vi "Oven Average of all temp.vi"() -> ()   [LabVIEW 2013, in "Generic Data Logger.lvlib" / "Fluke 2625A (Hydra II).lvlib" / "Fluke 2625A (Hydra II).lvclass"]
uses:
  Fluke 2625A (Hydra II).lvclass
  <vilib>/express/express shared/transition.llb/Dynamic To Waveform Array.vi
  <vilib>/express/express signal manip/GetorSetDDTAttributes/Set DDT Attributes/SetT0.vi
  <vilib>/express/express shared/transition.llb/Waveform Array To Dynamic.vi
  <vilib>/express/express signal manip/GetorSetDDTAttributes/Set DDT Attributes/Set DDT Properties.xnode
  <instrlib>/Fluke 2625A/Fluke 2625A.lvlib
  Data Logger/Data Logger.lvclass
panel:
  out "time delay":dbl
  out "min length":i32
  out "size(s) 2":i32
  out "before write":errorcluster
  out "error out":errorcluster
  out "Path":string
  out "selected path":path
  out "Current Average":dbl
  out "addign all values":dbl
  out "size(s)":i32
  out "length of stuff":i32
  out "String Array":string[](array[string])
  out "i":i32
  out "Numeric Array":dbl[](array[numeric])
  out "Raw String":string
  in  "Stop Button":bool
  in  "VISA resource name":refnum<visa-resource-name>
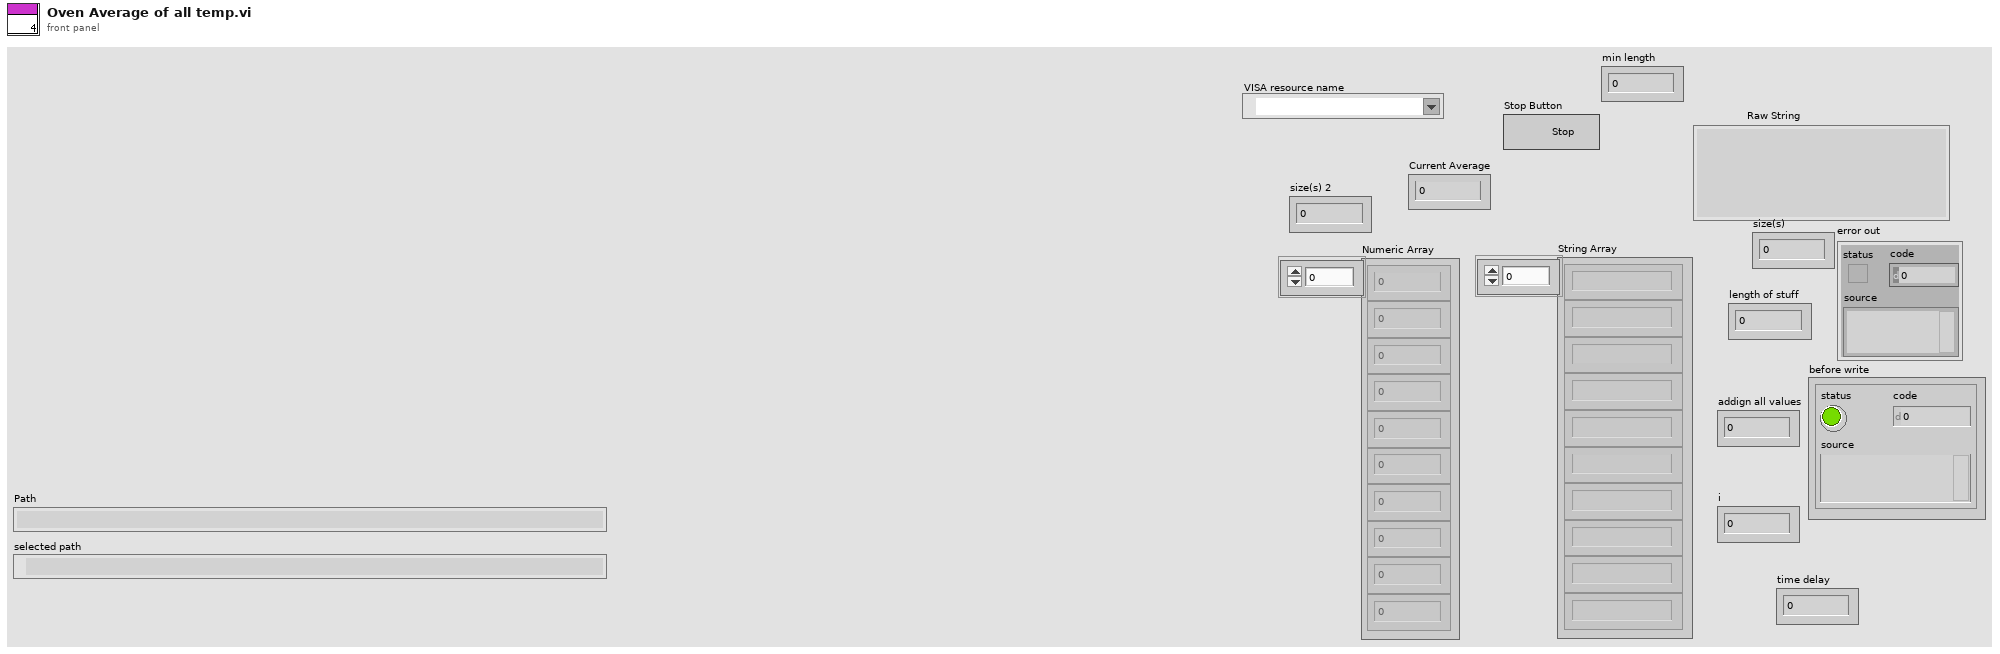
[diagram p1: front panel]
types:
  T1 = cluster{"Project Number":string, "Manufacturer":string, "Model":string, "Serial":string, "Comment":string}
  T2 = typedef "Generic Data Logger.lvlib/Fluke 2625A (Hydra II).lvlib/Fluke 2625A (Hydra II).lvclass/Unit Measurement.ctl" = cluster{"Function (5: Temp)":u16, "Channel":i8, "Thermocouple Type (0: J) 2":u16, "Name":string}
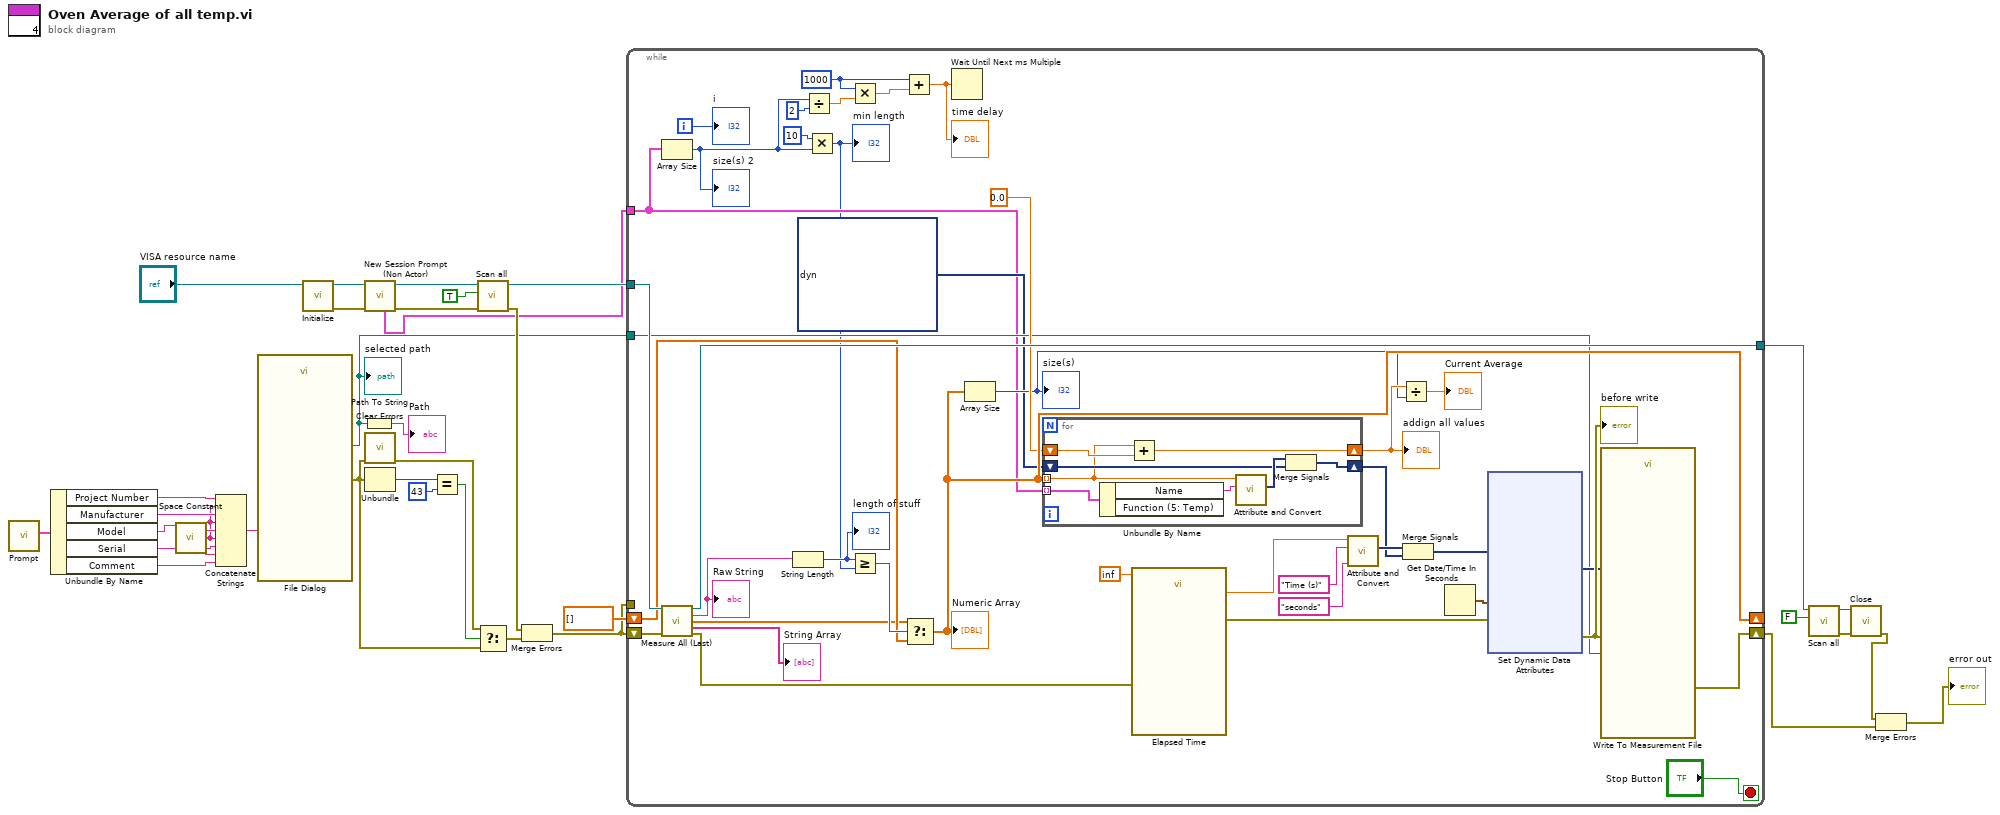
[diagram p0: block diagram]
diagram:
  n1 = call "Prompt.vi"() -> ("Cluster"=w26:T1)  [unwired: 11 in]
  n2 = Unbundle By Name(w26) -> ("Project Number"=w25:string, "Manufacturer"=w24:string, "Model"=w23:string, "Serial"=w22:string, "Comment"=w21:string)
  n3 = call <vilib>:"Space Constant.vi"() -> ("String"=w20:string)
  n4 = Concatenate Strings(w25, w20, w24, w20, w23, w20, w22, w20, w21) -> (w19:string)
  n5 = call "File Dialog"("default name"=w19) -> ("selected path"=w10:path, "error out"=w13:errorcluster)  [unwired: 11 in, 2 out]
  "selected path" <- w10
  n6 = call <instrlib>:"Initialize.vi"("VISA resource name"="VISA resource name") -> ("error out"=w33:errorcluster, "VISA resource name out"=w34:refnum<visa-resource-name>)  [unwired: 8 in, 1 out]
  n7 = Path To String(path=w10) -> (string=→"Path":string)
  n8 = call "New Session Prompt (Non Actor).vi"("error in (no error)"=w33, "VISA resource name"=w34) -> ("error out"=w29:errorcluster, "VISA resource name out"=w30:refnum<visa-resource-name>, "Array 2"=w9:T2[])  [unwired: 5 in, 2 out]
  n9 = call <vilib>:"Clear Errors.vi"("error in (no error)"=w13) -> ("error out"=w14:errorcluster)  [unwired: 6 in]
  n10 = Unbundle(w13) -> ("code"=w17:i32)  [unwired: 2 out]
  n11 = Equal?(x=w17, y=43) -> (x = y?=w15:bool)
  n12 = call <instrlib>:"Scan all.vi"("error in (no error)"=w29, "Start/Stop"=TRUE, "VISA resource name"=w30) -> ("error out"=w12:errorcluster, "VISA resource name out"=w28:refnum<visa-resource-name>)  [unwired: 7 in]
  n13 = Select(t=w14, s=w15, f=w13) -> (s? t:f=w11:errorcluster)
  n14 = Merge Errors(w12, w11) -> (w4:errorcluster)
  n15 = while {
    tunnel: w28 -> [w74]
    tunnel: w4 -> [_]
    tunnel: [w73] -> w6
    shift-right: [w65] -> _
    shift-left: dbl[] [] ("Numeric Array") -> [w66]
    tunnel: w10 -> [w54]
    tunnel: w9 -> [w43]
    shift-right: [w55] -> w2
    shift-left: w4 -> [w45]
    i -> [w71]
    stop <- "Stop Button" stop-if-true
    w37 = u32 1000 ("millisecond multiple")
    n16 = Array Size(array=w43) -> (size(s)=w40:i32)
    "size(s) 2" <- w40
    n17 = call <instrlib>:"Measure All (Last).vi"("VISA resource name out"=w74, "error in (no error)"=w45) -> ("VISA resource name out 2"=w73:refnum<visa-resource-name>, "Raw String"=w69:string, "Numeric Array"=w44:dbl[], "String Array"=→"String Array":string[], "error out 2"=w51:errorcluster)  [unwired: 9 in]
    "Raw String" <- w69
    n18 = String Length(string=w69) -> (length=w68:i32)
    "length of stuff" <- w68
    n19 = Divide(x=w40, y=2) -> (x/y=w36:dbl)
    n20 = Multiply(x=10 ("y"), y=w40) -> (x*y=w41:i32)
    "min length" <- w41
    n21 = Multiply(x=w37, y=w36) -> (x*y=w35:dbl)
    n22 = Greater Or Equal?(x=w68, y=w41) -> (x >= y?=w67:bool)
    n23 = Add(x=w37, y=w35) -> (x+y=w38:dbl)
    "time delay" <- w38
    n24 = Select(t=w44, s=w67, f=w66) -> (s? t:f=w65:dbl[])
    "Numeric Array" <- w65
    n25 = Wait Until Next ms Multiple(millisecond multiple=w38) -> ()  [unwired: 1 out]
    n26 = Array Size(array=w65) -> (size(s)=w62:i32)
    "size(s)" <- w62
    n27 = for {
      tunnel: w65 -> [w89] mode=indexing
      shift-right: [w90] -> w63
      shift-left: 0.0 ("read buffer") -> [w91]
      tunnel: w43 -> [w96] mode=indexing
      shift-right: [w92] -> w47
      shift-left: dynamicdata [] ("Waveform Graph") -> [w93]
      n28 = Unbundle By Name(w96) -> ("Name"=w95:string)  [unwired: 1 out]
      n29 = Add(x=w89, y=w91) -> (x+y=w90:dbl)
      n30 = call "Attribute and Convert.vi"("Signal Name"=w95, "Number in"=w89) -> ("Dynamic Signal Out"=w94:dynamicdata)  [unwired: 9 in]
      n31 = Merge Signals(w94, w93) -> (w92:dynamicdata)
    }
    "addign all values" <- w63
    n32 = call "Elapsed Time"("Time Target (s)"=inf, "error in (no error)"=w51) -> ("Elapsed Time (s)"=w52:dbl, "error out"=w50:errorcluster)  [unwired: 10 in, 6 out]
    n33 = call "Attribute and Convert.vi"("Unit"="seconds", "Signal Name"="Time (s)", "Number in"=w52) -> ("Dynamic Signal Out"=w48:dynamicdata)  [unwired: 8 in]
    n34 = Divide(x=w63, y=w62) -> (x/y=→"Current Average":dbl)
    n35 = Merge Signals(w48, w47) -> (w46:dynamicdata)
    n36 = Get Date/Time In Seconds() -> (seconds since 1Jan1904=w57:timestamp)
    n37 = xnode "Set Dynamic Data Attributes"("Signals In"=w46, "Timestamp"=w57, "error in"=w50) -> ("Signals Out"=w56:dynamicdata, "error out"=w58:errorcluster)  [unwired: 1 in]
    "before write" <- w58
    n38 = call "Write To Measurement File"("Signals"=w56, "error in (no error)"=w58, "Filename"=w54) -> ("error out"=w55:errorcluster)  [unwired: 14 in, 2 out]
    "i" <- w71
  }
  n39 = call <instrlib>:"Scan all.vi"("Start/Stop"=FALSE, "VISA resource name"=w6) -> ("error out"=w7:errorcluster, "VISA resource name out"=w8:refnum<visa-resource-name>)  [unwired: 8 in]
  n40 = call <instrlib>:"Close.vi"("error in (no error)"=w7, "VISA resource name"=w8) -> ("error out"=w3:errorcluster)  [unwired: 9 in]
  n41 = Merge Errors(w3, w2) -> (→"error out":errorcluster)
